vi "Arcade Drive Outputs Calculations.vi"(5 "Square Input":bool=TRUE, 6 "Turning Rate":dbl, 7 "Speed Rate":dbl, 8 "Turning Left & Right (Right Joystick)":dbl min=-1.0 max=1.0 step=0.1, 11 "Speed Forward & Reverse (Left JoysticK)":dbl min=-1.0 max=1.0 step=0.1) -> (2 "Right Motor":dbl, 3 "Left Motor":dbl)   [LabVIEW 2017]
panel:
  in  "Min Deadband":dbl
  in  "Max Deadband":dbl
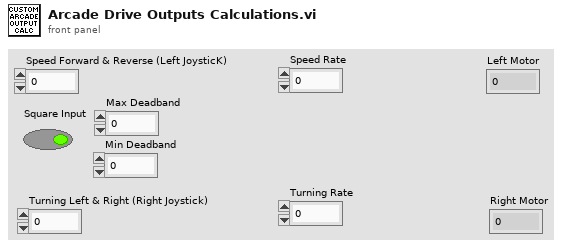
[diagram p1: front panel]
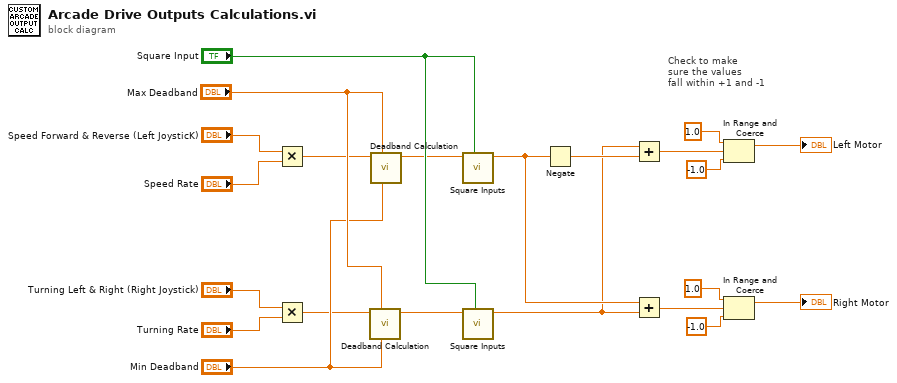
[diagram p0: block diagram]
diagram:
  # "Check to make\nsure the values\nfall within +1 and -1"
  n1 = Multiply(x="Speed Forward & Reverse (Left JoysticK)", y="Speed Rate") -> (x*y=w3:dbl)
  n2 = Multiply(x="Turning Left & Right (Right Joystick)", y="Turning Rate") -> (x*y=w2:dbl)
  n3 = call "Deadband Calculation.vi"("Min Deadband"="Min Deadband", "Max Deadband"="Max Deadband", "Deadband Check Input"=w2) -> ("Deadband Check Output"=w1:dbl)  [unwired: 8 in]
  n4 = call "Deadband Calculation.vi"("Min Deadband"="Min Deadband", "Max Deadband"="Max Deadband", "Deadband Check Input"=w3) -> ("Deadband Check Output"=w4:dbl)  [unwired: 8 in]
  n5 = call "Square Inputs.vi"("Square Input"="Square Input", "Joystick Input"=w4) -> ("Joystick Output"=w21:dbl)  [unwired: 9 in]
  n6 = call "Square Inputs.vi"("Square Input"="Square Input", "Joystick Input"=w1) -> ("Joystick Output"=w20:dbl)  [unwired: 9 in]
  n7 = Negate(x=w21) -> (-x=w22:dbl)
  n8 = Add(x=w20, y=w22) -> (x+y=w9:dbl)
  n9 = Add(x=w21, y=w20) -> (x+y=w10:dbl)
  n10 = In Range and Coerce(upper limit=1.0, x=w9, lower limit=-1.0) -> (coerced(x)=→"Left Motor":dbl)  [unwired: 1 out]
  n11 = In Range and Coerce(upper limit=1.0, x=w10, lower limit=-1.0) -> (coerced(x)=→"Right Motor":dbl)  [unwired: 1 out]
